vi "System-ExecInfo-Host.vi"() -> ()   [LabVIEW 2016]
uses:
  <vilib>/Powertrain Controls/Device Drivers/DCM/Rev0/RT/System ADC.ctl
  <vilib>/Powertrain Controls/Device Drivers/DCM/Rev0/RT/Internal Fault.ctl
  <vilib>/Powertrain Controls/Device Drivers/DCM/Rev0/RT/DCM - RT.lvclass
panel:
  in  "Reboot":bool
  out "IP_Address":string
  out "TargetName":string
  out "CalLoading":bool
  out "SCMInitError":bool
  out "FPGA_1_Error":bool
  out "App_Run_Time":sgl caption="[sec]"
  in  "_Hidden":enum32{"Page 1"}(tab)
  out "State":T3 caption="DCM System State" {"System ADC"."Fan [V]" format="%#_3p"; "System ADC"."Primary B1B2 [V]" format="%#_3p"; "System ADC"."Primary B3B4 [V]" format="%#_3p"; "System ADC"."Primary A3A4 [V]" format="%#_3p"; "System ADC"."Primary A1A2 [V]" format="%#_3p"; "System ADC"."MPRD [V]" format="%#_3p"; "System ADC"."Ext HV B [V]" format="%#_3p"; "System ADC"."Ext HV A [V]" format="%#_3p"; "System ADC"."Pump Zener B [V]" format="%#_3p"; "System ADC"."Pump Zener A [V]" format="%#_3p"; "System ADC"."DI Zener B [V]" format="%#_3p"; "System ADC"."DI Zener A [V]" format="%#_3p"; "System ADC"."Key [V]" format="%#_3p"; "System ADC"."DRVP [V]" format="%#_3p"; "System ADC"."Battery [V]" format="%#_3p"; "System ADC"."FET Driver [V]" format="%#_3p"; "System ADC"."Secondary B1B2 [V]" format="%#_3p"; "System ADC"."Secondary B3B4 [V]" format="%#_3p"; "System ADC"."Secondary A3A4 [V]" format="%#_3p"; "System ADC"."Secondary A1A2 [V]" format="%#_3p"; "System ADC"."Primary Range [V]" format="%#_3p"; "System ADC"."Temp Boost B [C]" format="%#_3p"; "System ADC"."Temp Primary A [C]" format="%#_3p"; "System ADC"."Temp Secondary A [C]" format="%#_3p"; "System ADC"."Temp Fan Intake [C]" format="%#_3p"; "System ADC"."Temp CPU [C]" format="%#_3p"; "System ADC"."Temp DI Zener B [C]" format="%#_3p"; "System ADC"."Temp DI B [C]" format="%#_3p"; "System ADC"."Temp DI Zener A [C]" format="%#_3p"; "System ADC"."Temp DI A [C]" format="%#_3p"; "System ADC"."Temp HH 7-12 [C]" format="%#_3p"; "System ADC"."Temp HH 1-6 [C]" format="%#_3p"; "System ADC"."AI 12 [V]" format="%#_3p"; "System ADC"."AI 11 [V]" format="%#_3p"; "System ADC"."AI 10 [V]" format="%#_3p"; "System ADC"."AI 9 [V]" format="%#_3p"; "System ADC"."AI 8 [V]" format="%#_3p"; "System ADC"."AI 7 [V]" format="%#_3p"; "System ADC"."AI 6 [V]" format="%#_3p"; "System ADC"."AI 5 [V]" format="%#_3p"; "System ADC"."AI 4 [V]" format="%#_3p"; "System ADC"."AI 3 [V]" format="%#_3p"; "System ADC"."AI 2 [V]" format="%#_3p"; "System ADC"."AI 1 [V]" format="%#_3p"}
  in  "Engine_Time_Reset":bool
  out "Time_Since_Start":sgl caption="[sec]"
  out "Engine_Time":sgl caption="[hr]"
  out "SysLoopError":errorcluster caption="System Loop Error"
  out "CmdLoopError":errorcluster caption="Command Loop Error"
  in  "SystemLoopPeriod_Set":u32 caption="[]"
  out "SystemLoopDuration":u32(slide) caption="[]"
  out "SystemLoopPeriod":u32 caption="[]"
  in  "CmdLoopPeriod_Set":u32 caption="[usec]"
  out "Engine_Out_Duration":u32(slide) caption="[]"
  out "Control_Duration":u32(slide) caption="[]"
  out "Engine_In_Duration":u32(slide) caption="[]"
  out "Hardware_Duration":u32(slide) caption="[usec]"
  out "CmdLoopDuration":u32(slide) caption="[]"
  out "CmdLoopPeriod":u32 caption="[usec]"
  out "Total_Mem":sgl(slide) caption="[bytes]"
  out "Memory_Used":sgl(slide) caption="[]"
  out "CPU_Load_TimeCrit":sgl(slide) caption="[]" scale=0.0..100.0
  out "CPU_Load":sgl(slide) caption="[%]" scale=0.0..100.0
  out "Storage_Space":u32(slide) caption="[]"
  out "Storage_Space_Used":u32(slide) caption="[]"
  # "Engine"
  # "Software"
  # "of"
  # "of"
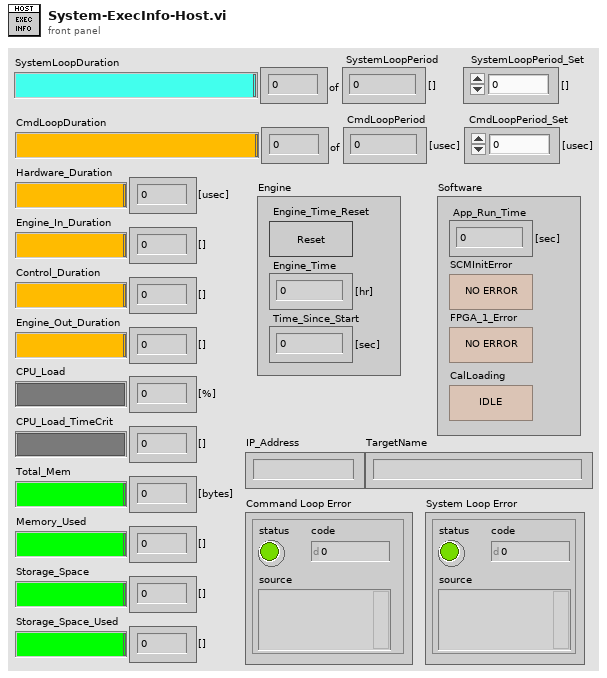
[diagram p1: front panel]
types:
  T1 = typedef "DCM - RT.lvclass/System ADC.ctl" = cluster{"AI 1 [V]":sgl, "AI 2 [V]":sgl, "AI 3 [V]":sgl, "AI 4 [V]":sgl, "AI 5 [V]":sgl, "AI 6 [V]":sgl, "AI 7 [V]":sgl, "AI 8 [V]":sgl, "AI 9 [V]":sgl, "AI 10 [V]":sgl, "AI 11 [V]":sgl, "AI 12 [V]":sgl, "Temp HH 1-6 [C]":sgl, "Temp HH 7-12 [C]":sgl, "Temp DI A [C]":sgl, "Temp DI Zener A [C]":sgl, "Temp DI B [C]":sgl, "Temp DI Zener B [C]":sgl, "Temp CPU [C]":sgl, "Temp Fan Intake [C]":sgl, "Temp Secondary A [C]":sgl, "Temp Primary A [C]":sgl, "Temp Boost B [C]":sgl, "Primary Range [V]":sgl, "Primary A1A2 [V]":sgl, "Primary A3A4 [V]":sgl, "Primary B3B4 [V]":sgl, "Primary B1B2 [V]":sgl, "Secondary A1A2 [V]":sgl, "Secondary A3A4 [V]":sgl, "Secondary B3B4 [V]":sgl, "Secondary B1B2 [V]":sgl, "Ext HV A [V]":sgl, "Ext HV B [V]":sgl, "FET Driver [V]":sgl, "Fan [V]":sgl, "Battery [V]":sgl, "DRVP [V]":sgl, "Key [V]":sgl, "DI Zener A [V]":sgl, "DI Zener B [V]":sgl, "Pump Zener A [V]":sgl, "Pump Zener B [V]":sgl, "MPRD [V]":sgl}
  T2 = typedef "DCM - RT.lvclass/Internal Fault.ctl" = enum32{"None", "Temp HH 1-6", "Temp HH 7-12", "Temp DI A", "Temp DI Zener A", "Temp DI B", "Temp DI Zener B", "Temp Intake", "Temp Primary A", "Temp Secondary A", "Temp Boost B", "Temp CPU", "Low Battery", "Inrush Protection", "A Run Enable", "B Run Enable", "Fan Speed"}
  T3 = cluster{"System ADC":T1, "IO Lock":bool, "HH Mode Config Error":bool, "Fan Speed 1 [RPM]":sgl, "Fan Speed 2 [RPM]":sgl, "Firmware Major Rev":u16, "Firmware Minor Rev":u16, "Internal Fault":T2, "Fault Value":dbl}
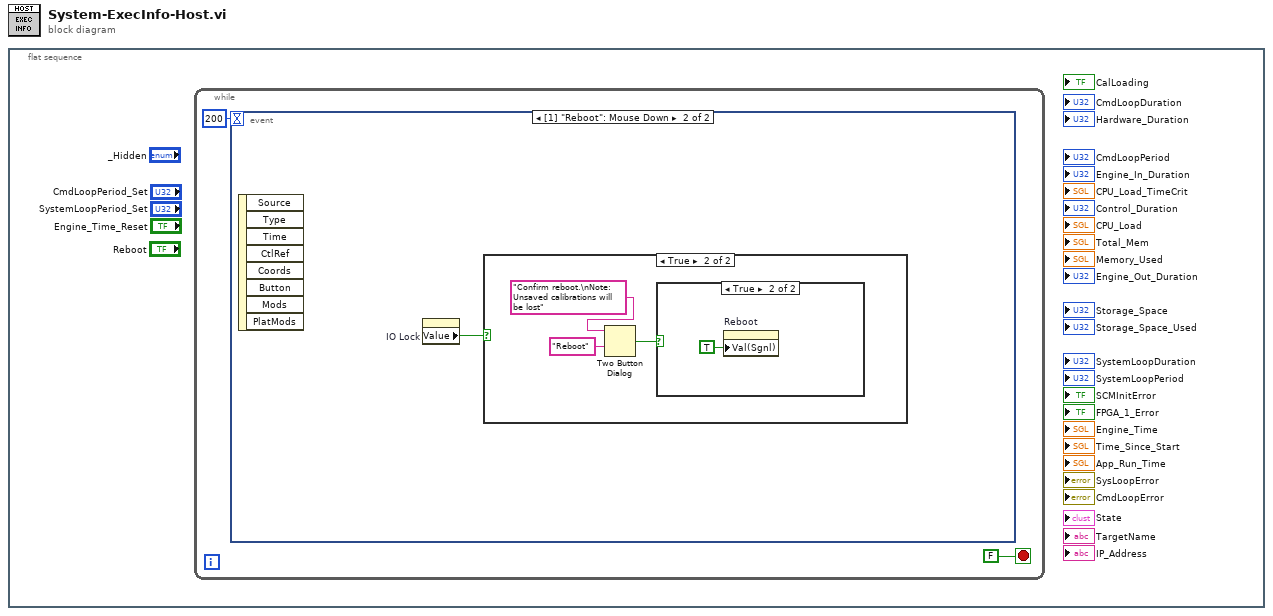
[diagram p0: block diagram]
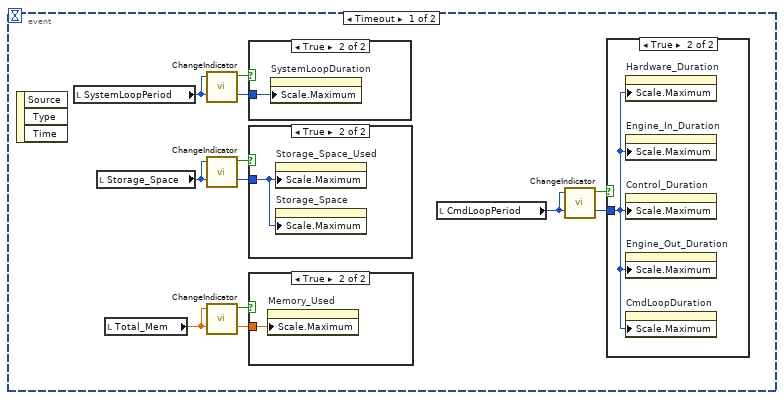
[diagram p2: hidden frame]
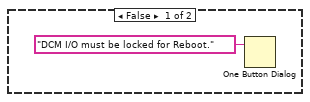
[diagram p7: hidden frame]
diagram:
  n1 = flat-sequence {
    frame #0 {
      n2 = while {
        stop <- FALSE stop-if-true
        n3 = event shown="[1] \"Reboot\": Mouse Down" {
          selector: _ -> [_ _]
          dyn-events: _ -> [_ _]
          timeout: 200 -> [_ _]
          event Timeout {
            n4 = event-data() -> ()  [unwired: 1 in, 3 out]
            n5 = local read "SystemLoopPeriod"() -> (w10:u32)
            n6 = local read "Storage_Space"() -> (w5:u32)
            n7 = local read "Total_Mem"() -> (w8:sgl)
            n8 = call "ChangeIndicator.vi"("Input"=w10) -> ("Change"=w9:bool)  [unwired: 9 in]
            n9 = call "ChangeIndicator.vi"("Input"=w5) -> ("Change"=w6:bool)  [unwired: 9 in]
            n10 = call "ChangeIndicator.vi"("Input"=w8) -> ("Change"=w7:bool)  [unwired: 9 in]
            n11 = case shown="True" w9 {
              tunnel: w10 -> [_ w11]
              frame False {
              }
              frame True {
                n12 = property on="SystemLoopDuration" class="Slide (strict)"("Scale.Maximum"=w11) -> ()  [unwired: 2 in, 2 out]
              }
            }
            n13 = case shown="True" w6 {
              tunnel: w5 -> [_ w13]
              frame False {
              }
              frame True {
                n14 = property on="Storage_Space_Used" class="Slide (strict)"("Scale.Maximum"=w13) -> ()  [unwired: 2 in, 2 out]
                n15 = property on="Storage_Space" class="Slide (strict)"("Scale.Maximum"=w13) -> ()  [unwired: 2 in, 2 out]
              }
            }
            n16 = case shown="True" w7 {
              tunnel: w8 -> [_ w12]
              frame False {
              }
              frame True {
                n17 = property on="Memory_Used" class="Slide (strict)"("Scale.Maximum"=w12) -> ()  [unwired: 2 in, 2 out]
              }
            }
            n18 = local read "CmdLoopPeriod"() -> (w4:u32)
            n19 = call "ChangeIndicator.vi"("Input"=w4) -> ("Change"=w3:bool)  [unwired: 9 in]
            n20 = case shown="True" w3 {
              tunnel: w4 -> [_ w14]
              frame False {
              }
              frame True {
                n21 = property on="Hardware_Duration" class="Slide (strict)"("Scale.Maximum"=w14) -> ()  [unwired: 2 in, 2 out]
                n22 = property on="Engine_In_Duration" class="Slide (strict)"("Scale.Maximum"=w14) -> ()  [unwired: 2 in, 2 out]
                n23 = property on="Control_Duration" class="Slide (strict)"("Scale.Maximum"=w14) -> ()  [unwired: 2 in, 2 out]
                n24 = property on="Engine_Out_Duration" class="Slide (strict)"("Scale.Maximum"=w14) -> ()  [unwired: 2 in, 2 out]
                n25 = property on="CmdLoopDuration" class="Slide (strict)"("Scale.Maximum"=w14) -> ()  [unwired: 2 in, 2 out]
              }
            }
          }
          event "Reboot": Mouse Down {
            n26 = event-data() -> ()  [unwired: 1 in, 8 out]
            n27 = property on="IO Lock" class="Bool (strict)"() -> ("Value"=w15:bool)  [unwired: 2 in, 2 out]
            n28 = case shown="True" w15 {
              frame False {
                n29 = One Button Dialog(message="DCM I/O must be locked for Reboot.") -> ()  [unwired: 1 in, 1 out]
              }
              frame True {
                n30 = Two Button Dialog(message="Confirm reboot.\nNote:  Unsaved calibrations will be lost", 2:"Reboot" ("T button name (\"OK\")")) -> (T button?=w19:bool)  [unwired: 1 in]
                n31 = case shown="True" w19 {
                  frame False {
                  }
                  frame True {
                    n32 = property on="Reboot" class="Bool (strict)"("Val(Sgnl)"=TRUE ("Value (Signaling)")) -> ()  [unwired: 2 in, 2 out]
                  }
                }
              }
            }
          }
        }
      }
    }
  }
